vi "SetPercentNeon.vi"(1 "data":dbl[](array[numeric]), 4 "NewVal":dbl, 5 "Old Value":dbl) -> (18 "Set Value":dbl)   [LabVIEW 2014, in "Panels.lvlib"]
uses:
  Panels.lvlib
  CSCore/CSSystem/CoreDefs/CoreDefs.call_type.ctl
  CSCore/BaseProcess/BaseProcess.descriptor string definition.ctl
  CSCore/CSSystem/CoreDefs/CoreDefs.rawDataType.ctl
  Instance           1 22Saved   SetPercentNeon .vi
  CSCore/CSSystem/CoreLib/CoreLib.short 2 byte array.vi
  CSCore/CSSystem/CoreLib/CoreLib.double 2 byte array.vi
  CSCore/CSSystem/CoreLib/CoreLib.string 2 byte array.vi
  CSCore/CSSystem/CoreLib/CoreLib.lvlib
  CSCore/BaseProcess/BaseProcess.lvlib
panel:
  in  "call cluster in":T1={"Object"="", "Selector"="", "CallType"=enum."synchronous", "Async Object"="", "Async Selector"="", "Data Descriptor"="", "Data"=[], "Error #"=0, "Expire"=0}
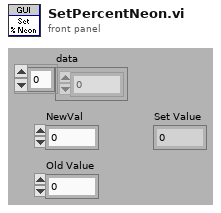
[diagram p1: front panel]
types:
  T1 = typedef "CoreDefs.call_type.ctl" = cluster{"Object":string, "Selector":string, "CallType":enum16{"simple", "synchronous", "asynchronous"}, "Async Object":string, "Async Selector":string, "Data Descriptor":T2, "Data":T3, "Error #":i32, "Expire":u32}
  T2 = typedef "BaseProcess.lvlib/BaseProcess.descriptor string definition.ctl" = string
  T3 = typedef "CoreDefs.rawDataType.ctl" = i8[]
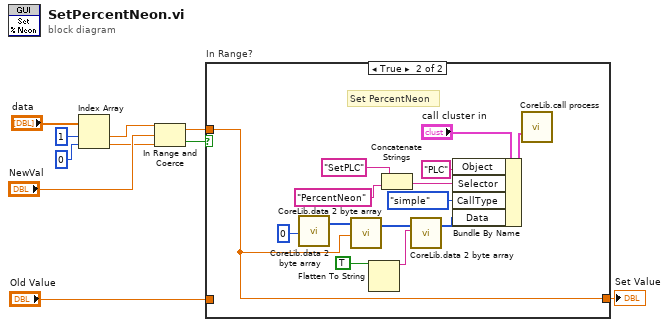
[diagram p0: block diagram]
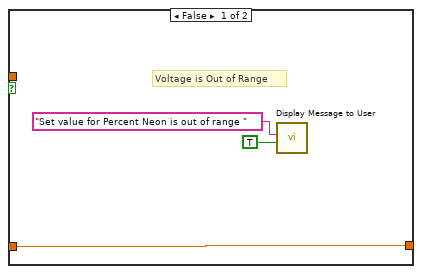
[diagram p2: hidden frame]
diagram:
  n1 = Index Array(array="data", index #1=1 ("index"), index #2=0 ("index")) -> (element #1=w8:dbl, element #2=w9:dbl)
  n2 = In Range and Coerce(upper limit=w8, x="NewVal", lower limit=w9) -> (coerced(x)=w3:dbl, In Range?=w4:bool)
  n3 = case "In Range?" shown="True" w4 {
    tunnel: w3 -> [_ w14]
    tunnel: [w11 w14] -> w2
    tunnel: "Old Value" -> [w11 _]
    frame False {
      # "Voltage is Out of Range"
      n4 = call "Display Message to User"("Enable"=TRUE, "Message"="Set value for Percent Neon is out of range " ("string")) -> ()  [unwired: 8 in, 2 out]
    }
    frame True {
      # "Set PercentNeon"
      n5 = call-poly "CoreLib.data 2 byte array.vi"("i16"=i16 0 ("f64")) -> ("byteArray out"=w27:T3)  [unwired: 18 in]
      n6 = call-poly "CoreLib.data 2 byte array.vi"("byteArray"=w27, "f64"=w14) -> ("byteArray out"=w22:T3)  [unwired: 17 in]
      n7 = Flatten To String(anything=TRUE) -> (data string=w23:string)  [unwired: 3 in, 2 out]
      n8 = Concatenate Strings("SetPLC" ("string"), "PercentNeon" ("string")) -> (w17:string)
      n9 = call-poly "CoreLib.data 2 byte array.vi"("byteArray"=w22, "string"=w23) -> ("byteArray out"=w25:T3)  [unwired: 17 in]
      n10 = Bundle By Name(cluster="call cluster in", "Object"="PLC", "Selector"=w17, "CallType"=enum16{"simple", "synchronous", "asynchronous"}."simple", "Data"=w25) -> (w20:T1)
      n11 = call "CoreLib.call process.vi"("call cluster in"=w20) -> ()  [unwired: 13 in, 2 out]
    }
  }
  "Set Value" <- w2
